vi "Stop_glob.vi"() -> ()   [LabVIEW 2024]
panel:
  out "Boolean 2":bool
  out "Boolean":bool
  in  "stop":bool
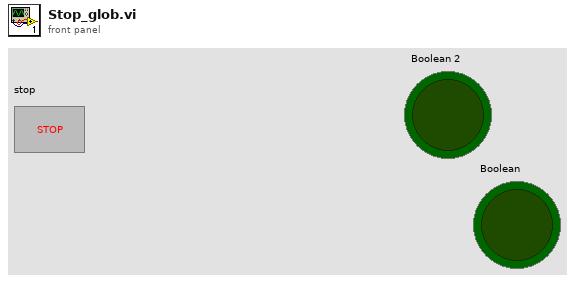
[diagram p1: front panel]
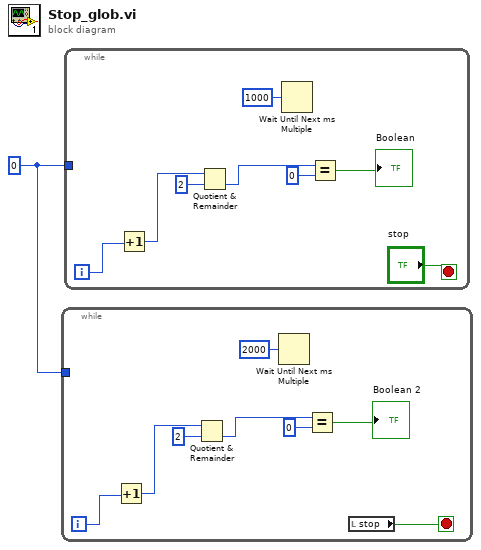
[diagram p0: block diagram]
diagram:
  w1 = 0
  n1 = while {
    tunnel: w1 -> [_]
    i -> [w8]
    stop <- w2 stop-if-true
    n2 = Increment(x=w8) -> (x+1=w7:i32)
    n3 = Quotient & Remainder(x=w7, y=2) -> (floor(x/y)=w5:i32)  [unwired: 1 out]
    n4 = Wait Until Next ms Multiple(millisecond multiple=u32 2000) -> ()  [unwired: 1 out]
    n5 = Equal?(x=w5, y=0) -> (x = y?=→"Boolean 2":bool)
    n6 = local read "stop"() -> (w2:bool)
  }
  n7 = while {
    tunnel: w1 -> [_]
    i -> [w15]
    stop <- "stop" stop-if-true
    n8 = Increment(x=w15) -> (x+1=w14:i32)
    n9 = Quotient & Remainder(x=w14, y=2) -> (floor(x/y)=w12:i32)  [unwired: 1 out]
    n10 = Wait Until Next ms Multiple(millisecond multiple=u32 1000) -> ()  [unwired: 1 out]
    n11 = Equal?(x=w12, y=0) -> (x = y?=→"Boolean":bool)
  }
